vi "config.vi"() -> ()   [LabVIEW 2016]
uses:
  <vilib>/Utility/config.llb/Read Key (Double).vi
  <vilib>/Utility/config.llb/Write Key (Double).vi
  <vilib>/Utility/config.llb/Write Key (I32).vi
  <vilib>/Utility/config.llb/NI_LVConfig.lvlib
panel:
  out "value":i32
  in  "configuration file path":path
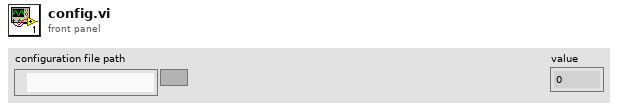
[diagram p1: front panel]
types:
  T1 = typedef "NI_LVConfig.lvlib/Config Data RefNum.ctl" = refnum<k1>
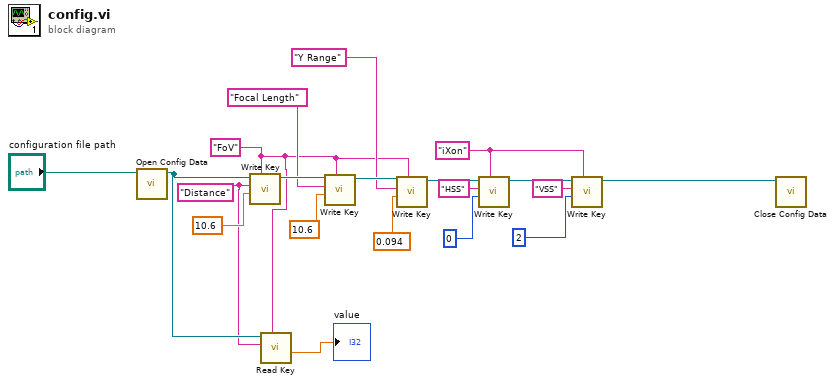
[diagram p0: block diagram]
diagram:
  w3 = "iXon" ("section")
  w9 = "Distance" ("key")
  w10 = "FoV" ("section")
  n1 = call <vilib>:"Open Config Data.vi"("configuration file path"="configuration file path") -> ("refnum"=w11:T1)  [unwired: 8 in, 2 out]
  n2 = call-poly <vilib>:"Write Key.vi"("section"=w10, "value"=10.6, "key"=w9, "refnum"=w11) -> ("refnum out"=w19:T1)  [unwired: 5 in, 2 out]
  n3 = call-poly <vilib>:"Read Key.vi"("section"=w10, "key"=w9, "refnum"=w11) -> ("value"=→"value":dbl)  [unwired: 5 in, 3 out]
  n4 = call-poly <vilib>:"Write Key.vi"("section"=w10, "value"=10.6, "key"="Focal Length", "refnum"=w19) -> ("refnum out"=w16:T1)  [unwired: 5 in, 2 out]
  n5 = call-poly <vilib>:"Write Key.vi"("section"=w10, "value"=0.094, "key"="Y Range", "refnum"=w16) -> ("refnum out"=w13:T1)  [unwired: 5 in, 2 out]
  n6 = call-poly <vilib>:"Write Key.vi"("section"=w3, "value"=0, "key"="HSS", "refnum"=w13) -> ("refnum out"=w7:T1)  [unwired: 5 in, 2 out]
  n7 = call-poly <vilib>:"Write Key.vi"("section"=w3, "value"=2, "key"="VSS", "refnum"=w7) -> ("refnum out"=w4:T1)  [unwired: 5 in, 2 out]
  n8 = call <vilib>:"Close Config Data.vi"("refnum"=w4) -> ()  [unwired: 9 in, 2 out]
